vi "SSL_get_error.vi"(8 "error in (no error)":errorcluster, 10 "SSL return code":i32, 11 "SSL-Lib in":refnum<class "SSL.lvclass">) -> (0 "error out":errorcluster, 2 "Error Code":u32, 3 "SSL-Lib out":refnum<class "SSL.lvclass">)   [LabVIEW 2013, in "SSL_Lib.lvlib" / "SSL.lvclass"]
uses:
  SSL.lvclass
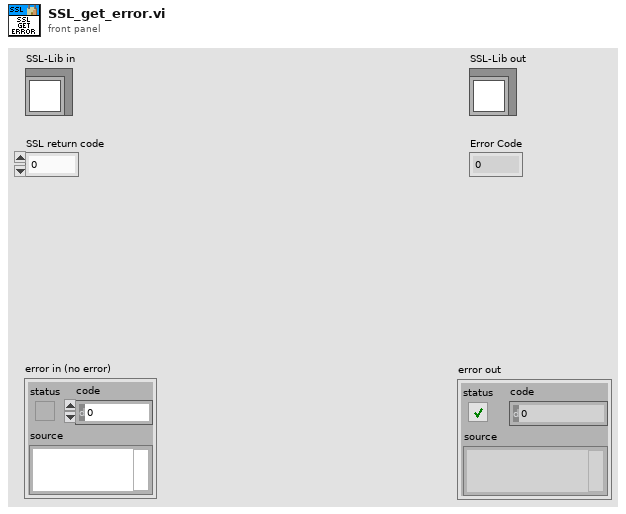
[diagram p1: front panel]
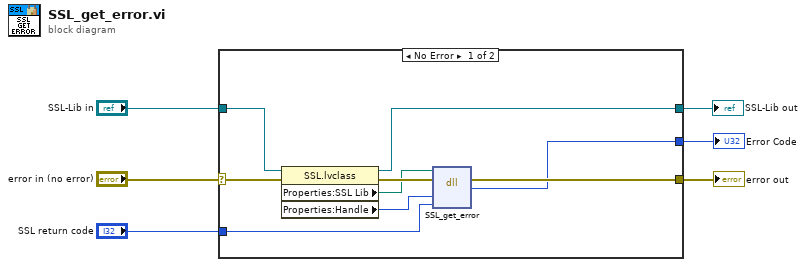
[diagram p0: block diagram]
diagram:
  n1 = case shown="No Error" "error in (no error)" {
    selector: "error in (no error)" -> [w15 w16]
    tunnel: [w8 w17] -> w4
    tunnel: "SSL-Lib in" -> [w7 w17]
    tunnel: "SSL return code" -> [w14 _]
    tunnel: [w13 w16] -> w2
    tunnel: [w12 _] -> w1
    frame No Error {
      n2 = property class="SSL.lvclass"(reference=w7, error in=w15) -> (reference out=w8:refnum<class "SSL.lvclass">, error out=w11:errorcluster, "Properties:SSL Lib"=w10:path, "Properties:Handle"=w9:u64)
      n3 = dll-call lib="C:/Program Files (x86)/National Instruments/Shared/nissl/NIssleay32.dll" fn="SSL_get_error"(path in=w10, error in=w11, "SSL"=w9, "ret"=w14) -> (error out=w13:errorcluster, "return type"=w12:u32)  [unwired: 3 in, 1 out]
    }
    frame Error {
    }
  }
  "SSL-Lib out" <- w4
  "error out" <- w2
  "Error Code" <- w1
